vi "Set_motor_direction_New.vi"(0 "TCP Network Connection in":refnum<k5>, 1 "Step status":bool, 5 "Step Count":i32, 7 "ADC distance":dbl, 9 "Possition selector":T1(radio), 11 "error in (no error)":errorcluster) -> (4 "TCP Network Connection out":refnum<k5>, 15 "error out":errorcluster)   [LabVIEW 2019]
panel:
  in  "ADC possitions":dbl[](array[numeric])=[6.31684, 27.7371, 181.99, 240.785, 293.499]
  in  "Step possitions":dbl[](array[numeric])=[-1280.0, -5428.0, -35785.0, -47327.0, -57601.0]
  out "Driver response":bool
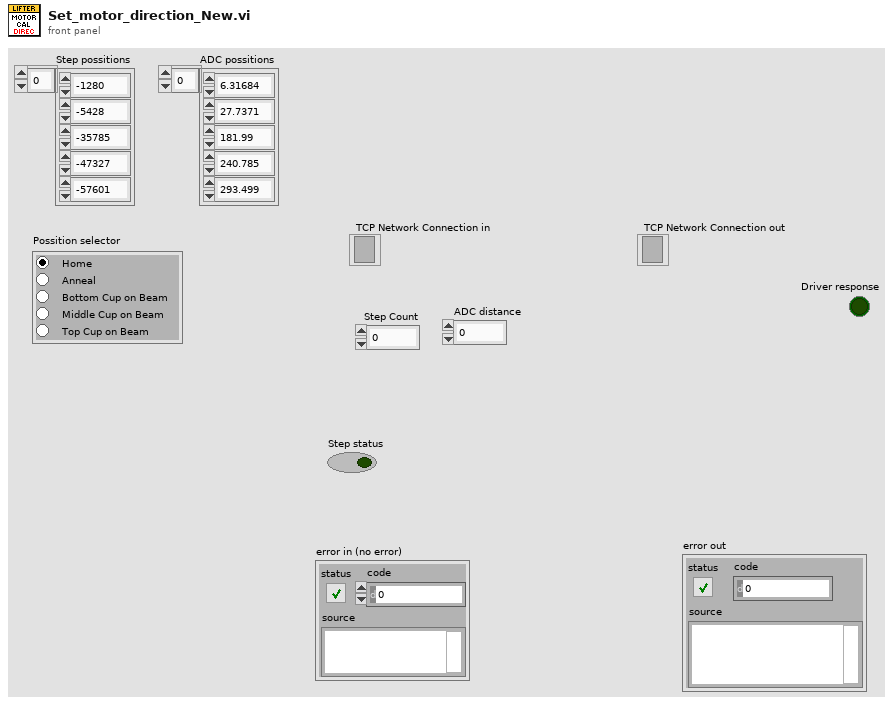
[diagram p1: front panel]
types:
  T1 = enum32{"Home", "Anneal", "Bottom Cup on Beam", "Middle Cup on Beam", "Top Cup on Beam"}
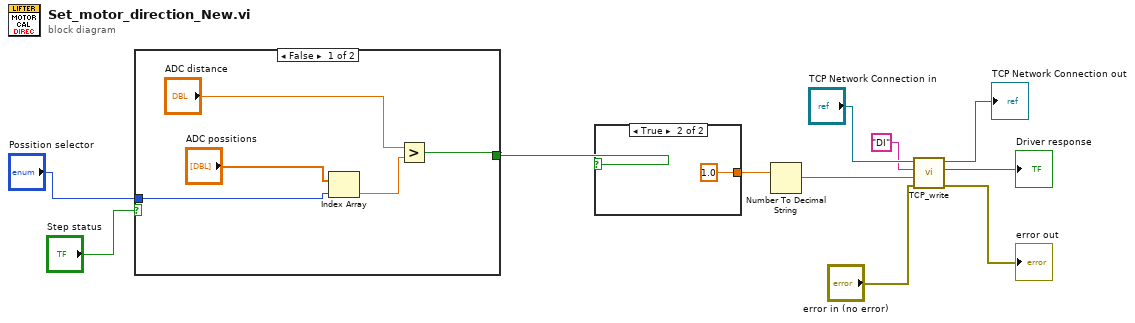
[diagram p0: block diagram]
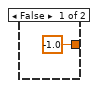
[diagram p2: hidden frame]
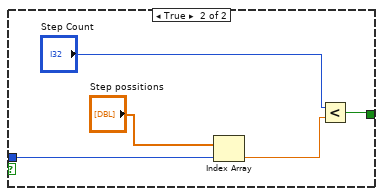
[diagram p3: hidden frame]
diagram:
  n1 = case shown="False" "Step status" {
    tunnel: [w15 w21] -> w11
    tunnel: "Possition selector" -> [w12 w18]
    frame False {
      n2 = Index Array(array="ADC possitions", index=w12) -> (element=w14:dbl)
      n3 = Greater?(x="ADC distance", y=w14) -> (0:w15:bool)
    }
    frame True {
      n4 = Index Array(array="Step possitions", index=w18) -> (element=w17:dbl)
      n5 = Less?(x="Step Count", y=w17) -> (x < y?=w21:bool)
    }
  }
  n6 = case shown="True" w11 {
    tunnel: [-1.0 ("Direction") 1.0 ("Direction")] -> w10
    frame False {
    }
    frame True {
    }
  }
  n7 = Number To Decimal String(number=w10) -> (decimal integer string=w7:string)  [unwired: 1 in]
  n8 = call "TCP_write.vi"("error in"="error in (no error)", "Parameter 2"=w7, "Parameter 1"="DI" ("string"), "connection ID"="TCP Network Connection in") -> ("error out"=→"error out":errorcluster, "Driver response"=→"Driver response":bool, "TCP Network Connection out"=→"TCP Network Connection out":refnum<k5>)  [unwired: 5 in]
